vi "CCM-Check Digital Output Lines.vi"(0 "TTL Devices":refnum<class "TTLControlledDevice.lvclass">[](array[class]), 5 "Tables":cluster{"Table":T1[]}[](array[cluster]), 9 "DI Port":string, 11 "error in (no error)":errorcluster, 12 "Buffered DO Port":string, 13 "DO Lines":string[](array[string])) -> (6 "Tables thru":cluster{"Table":T1[]}[](array[cluster]), 15 "error out":errorcluster)   [LabVIEW 2020]
uses:
  epl-tosca/LV Source/TTL VIs/Device Classes/Base Class/TTLControlledDevice.lvclass
  Type Defs/CM-Connection.ctl
  epl-tosca/LV Source/TTL VIs/Device Classes/Base Class/TTLControlledDevice.lvclass/TTLControlledDevice.ctl
  epl-tosca/LV Source/TTL VIs/Device Classes/Base Class/Read Line.vi
  epl-tosca/LV Source/TTL VIs/Device Classes/Base Class/Read Name.vi
  <vilib>/regexp/Match Regular Expression.xnode
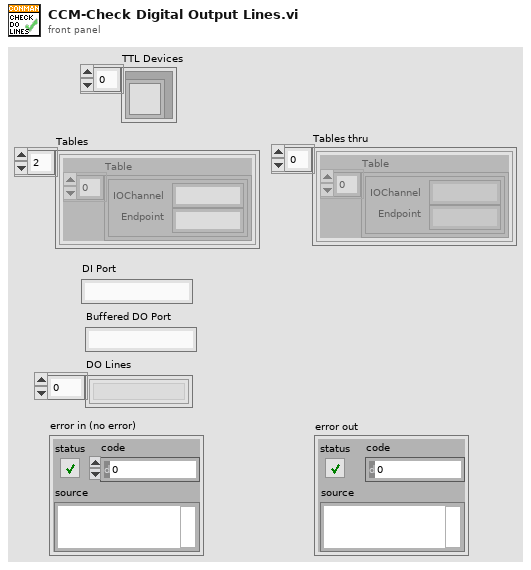
[diagram p1: front panel]
types:
  T1 = typedef "CM-Connection.ctl" = cluster{"IOChannel":string, "Endpoint":string}
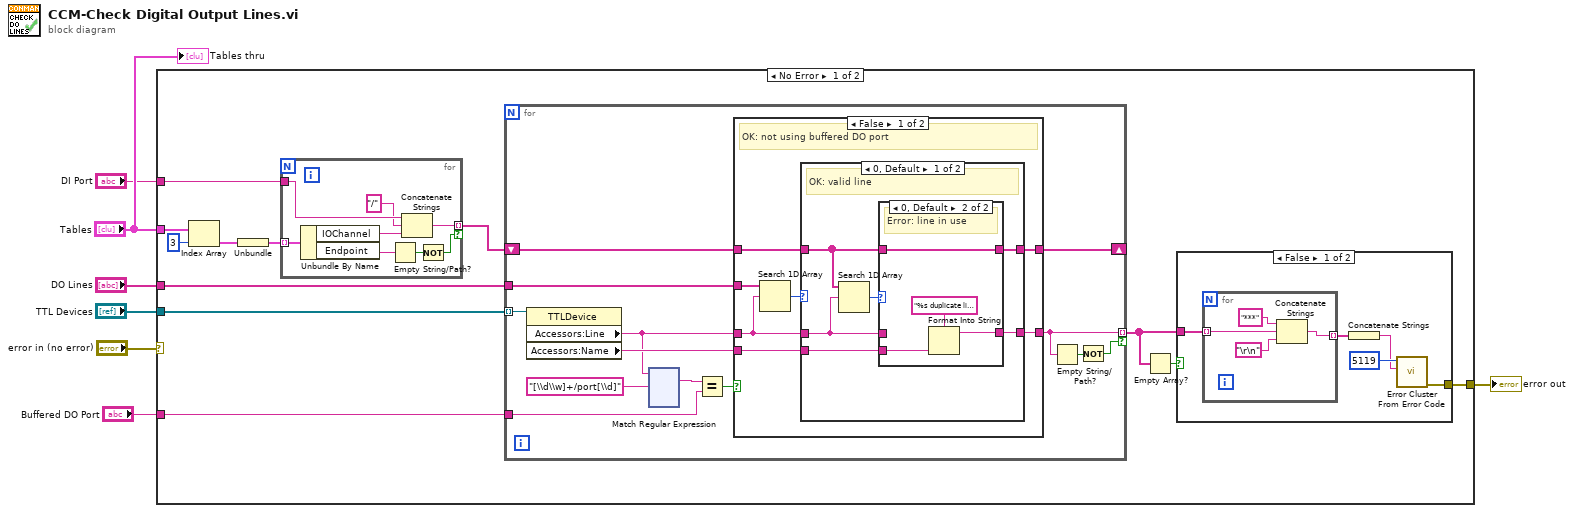
[diagram p0: block diagram]
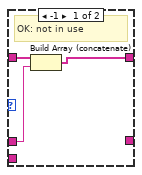
[diagram p2: hidden frame]
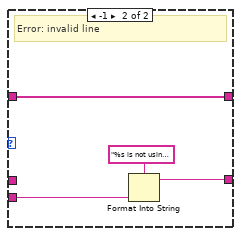
[diagram p3: hidden frame]
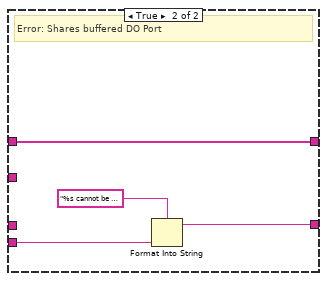
[diagram p4: hidden frame]
diagram:
  n1 = case shown="No Error" "error in (no error)" {
    selector: "error in (no error)" -> [_ w192]
    tunnel: [w18 w192] -> w7
    tunnel: "TTL Devices" -> [w17 _]
    tunnel: "Buffered DO Port" -> [w16 _]
    tunnel: "DO Lines" -> [w15 _]
    tunnel: "Tables" -> [w13 _]
    tunnel: "DI Port" -> [w9 _]
    frame No Error {
      n2 = Index Array(array=w13, index=3) -> (element=w11:cluster{"Table":T1[]})
      n3 = Unbundle(w11) -> ("Table"=w10:T1[])
      n4 = for {
        tunnel: w10 -> [w27] mode=indexing
        tunnel: w9 -> [w25]
        tunnel: [w23] -> w8 mode=indexing if=w20
        n5 = Unbundle By Name(w27) -> ("IOChannel"=w26:string, "Endpoint"=w22:string)
        n6 = Empty String/Path?(string/path=w22) -> (empty?=w21:bool)
        n7 = Concatenate Strings(w25, "/" ("string"), w26) -> (w23:string)
        n8 = Not(x=w21) -> (.not. x?=w20:bool)
      }
      n9 = for {
        tunnel: w17 -> [w40] mode=indexing
        shift-right: [w34] -> _
        shift-left: w8 -> [w37]
        tunnel: w16 -> [w38]
        tunnel: [w32] -> w14 mode=indexing if=w30
        tunnel: w15 -> [w33]
        n10 = property class="TTLDevice"(reference=w40) -> ("Accessors:Line"=w28:string, "Accessors:Name"=w35:string)  [unwired: 1 in, 2 out]
        n11 = xnode "Match Regular Expression"("input string"=w28, "regular expression"="[\\d\\w]+/port[\\d]") -> ("whole match"=w39:string)  [unwired: 4 in, 4 out]
        n12 = Equal?(x=w39, y=w38) -> (x = y?=w36:bool)
        n13 = case shown="False" w36 {
          tunnel: w37 -> [w161 w182]
          tunnel: w35 -> [w156 w180]
          tunnel: [w160 w182] -> w34
          tunnel: [w155 w179] -> w32
          tunnel: w28 -> [w158 _]
          tunnel: w33 -> [w159 _]
          frame False {
            # "OK: not using buffered DO port"
            n14 = Search 1D Array(1D array=w159, element=w158) -> (index of element=w157:i32)  [unwired: 1 in]
            n15 = case shown="0, Default" w157 {
              tunnel: w161 -> [w166 w178]
              tunnel: [w165 w178] -> w160
              tunnel: w158 -> [w164 _]
              tunnel: w156 -> [w163 w176]
              tunnel: [w162 w175] -> w155
              frame 0, Default {
                # "OK: valid line"
                n16 = Search 1D Array(1D array=w166, element=w164) -> (index of element=w167:i32)  [unwired: 1 in]
                n17 = case shown="0, Default" w167 {
                  tunnel: w166 -> [w170 w174]
                  tunnel: w164 -> [w169 _]
                  tunnel: [w168 w174] -> w165
                  tunnel: w163 -> [_ w172]
                  tunnel: [_ w171] -> w162
                  frame -1 {
                    # "OK: not in use"
                    n18 = Build Array (concatenate)(w170, w169) -> (w168:string[])
                  }
                  frame 0, Default {
                    # "Error: line in use"
                    n19 = Format Into String(format string="%s duplicate line selected", w172) -> (resulting string=w171:string)  [unwired: 2 in, 1 out]
                  }
                }
              }
              frame -1 {
                # "Error: invalid line"
                n20 = Format Into String(format string="%s is not using a valid digital line.", w176) -> (resulting string=w175:string)  [unwired: 2 in, 1 out]
              }
            }
          }
          frame True {
            # "Error: Shares buffered DO Port"
            n21 = Format Into String(format string="%s cannot be on the buffered DO port", w180) -> (resulting string=w179:string)  [unwired: 2 in, 1 out]
          }
        }
        n22 = Empty String/Path?(string/path=w32) -> (empty?=w31:bool)
        n23 = Not(x=w31) -> (.not. x?=w30:bool)
      }
      n24 = Empty Array?(array=w14) -> (empty?=w19:bool)
      n25 = case shown="False" w19 {
        tunnel: w14 -> [w185 _]
        tunnel: [w186 _] -> w18
        frame False {
          n26 = for {
            tunnel: w185 -> [w189] mode=indexing
            tunnel: [w190] -> w184 mode=indexing
            n27 = Concatenate Strings("***" ("string"), w189, "\r\n") -> (w190:string)
          }
          n28 = Concatenate Strings(w184) -> (w183:string)
          n29 = call <vilib>:"Error Cluster From Error Code.vi"("error message (\"\")"=w183, "error code (0)"=5119 ("specific error code to clear (0: all)")) -> ("error out"=w186:errorcluster)  [unwired: 7 in]
        }
        frame True {
        }
      }
    }
    frame Error {
    }
  }
  "error out" <- w7
  "Tables thru" <- "Tables"
